vi "Remove NaN in a 2D Array.vi"(8 "error in (no error)":errorcluster, 10 "Array in":dbl[][](array[numeric])=[[nan, 1.0, nan, 2.0, nan, 3.0, nan, 4.0]]) -> (0 "error out":errorcluster, 2 "Array out":dbl[][](array[numeric]))   [LabVIEW 2015, in "Zen Analytics.lvclass"]
doc: "Removes NaN in array."
uses:
  Zen Analytics.lvclass
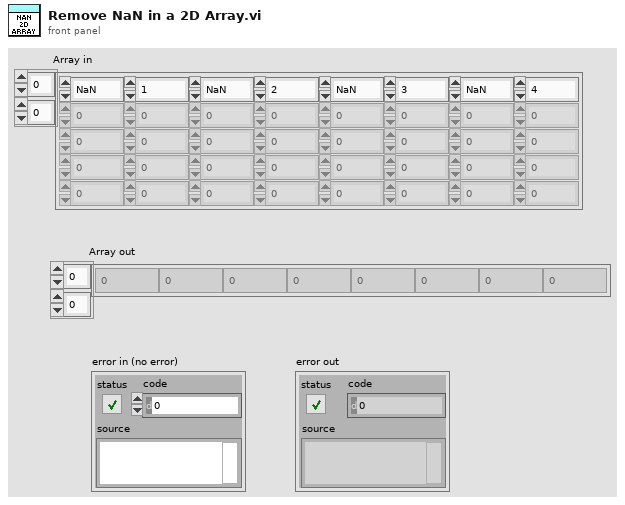
[diagram p1: front panel]
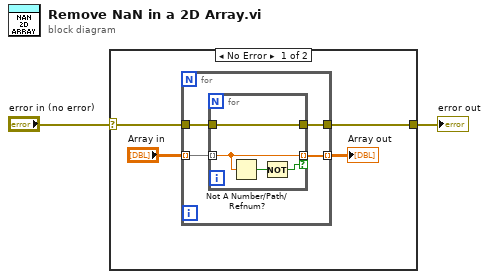
[diagram p0: block diagram]
diagram:
  n1 = case shown="No Error" "error in (no error)" {
    selector: "error in (no error)" -> [w4 w15]
    tunnel: [w3 w15] -> w1
    frame No Error {
      n2 = for {
        tunnel: "Array in" -> [w10] mode=indexing
        tunnel: [w9] -> w5 mode=indexing
        tunnel: w4 -> [w8]
        tunnel: [w7] -> w3
        n3 = for {
          tunnel: w10 -> [w14] mode=indexing
          tunnel: [w14] -> w9 mode=indexing if=w12
          tunnel: [w11] -> w7
          tunnel: w8 -> [w11]
          n4 = Not A Number/Path/Refnum?(number/path/refnum=w14) -> (NaN/Path/Refnum?=w13:bool)
          n5 = Not(x=w13) -> (.not. x?=w12:bool)
        }
      }
      "Array out" <- w5
    }
    frame Error {
    }
  }
  "error out" <- w1
